vi "Wait For Deploy.vi"(11 "NetCPU in":refnum<class "NetCPU.lvclass">) -> (0 "deployed":bool, 3 "NetCPU out":refnum<class "NetCPU.lvclass">)   [LabVIEW 2020, in "NI_TargetHelper.lvlib" / "NetCPU.lvclass"]
uses:
  <vilib>/TargetSupport/NI_TargetHelper/NetCPU/NetCPU.lvclass
  <vilib>/TargetSupport/NI_TargetHelper/NetCPU/NetCPU.lvclass/NetCPU.ctl
  <vilib>/TargetSupport/NI_TargetHelper/Instance VIref.ctl
  <vilib>/TargetSupport/NI_TargetHelper/NI_TargetHelper.lvlib
panel:
  out "error out":errorcluster
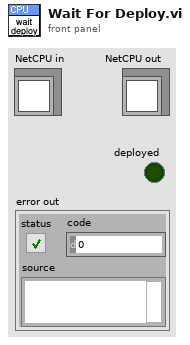
[diagram p1: front panel]
types:
  T1 = typedef "NI_TargetHelper.lvlib/Instance VIref.ctl" = refnum<vi>
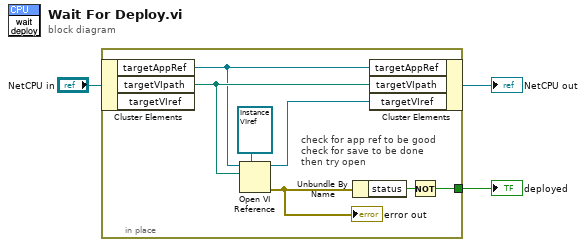
[diagram p0: block diagram]
diagram:
  n1 = in-place {
    in-place-border: [w6] -> w1
    # "check for app ref to be good\ncheck for save to be done\nthen try open"
    n2 = in-place-cluster #1("NetCPU in") -> ("targetAppRef"=w7:refnum<vi>, "targetVIpath"=w8:path)  [unwired: 1 out]
    n3 = Open VI Reference(type specifier VI Refnum (for type only)=T1 refnum ("targetVIref"), application reference (local)=w7, vi path=w8) -> (vi reference=w5:T1, error out=w10:errorcluster)  [unwired: 3 in]
    "error out" <- w10
    n4 = Unbundle By Name(w10) -> ("status"=w9:bool)
    n5 = in-place-cluster #1("targetAppRef"=w7, "targetVIpath"=w8, "targetVIref"=w5) -> (→"NetCPU out":refnum<class "NetCPU.lvclass">)
    n6 = Not(x=w9) -> (.not. x?=w6:bool)
  }
  "deployed" <- w1
